vi "读取数据库.vi"(5 "精度(6)":i16=2, 7 "condition":string, 8 "error in (no error)":errorcluster caption="错误输入（无错误）", 9 "database":string="database1.mdb", 10 "显示项":string[](array[string]), 11 "组合框":string(combo)) -> (0 "error out":errorcluster caption="错误输出", 1 "columns":string[](array[string]), 2 "data":variant[][](array[variant]), 3 "表格":string[][](table))   [LabVIEW 2016]
uses:
  <vilib>/Utility/sysdir.llb/System Directory Type.ctl
  <vilib>/addons/database/Connection.llb/DB Tools Open Connec (String).vi
  <vilib>/addons/database/_DB Variant To Data/Database Variant To Data.xnode
  <vilib>/addons/database/NI_Database_API.lvlib
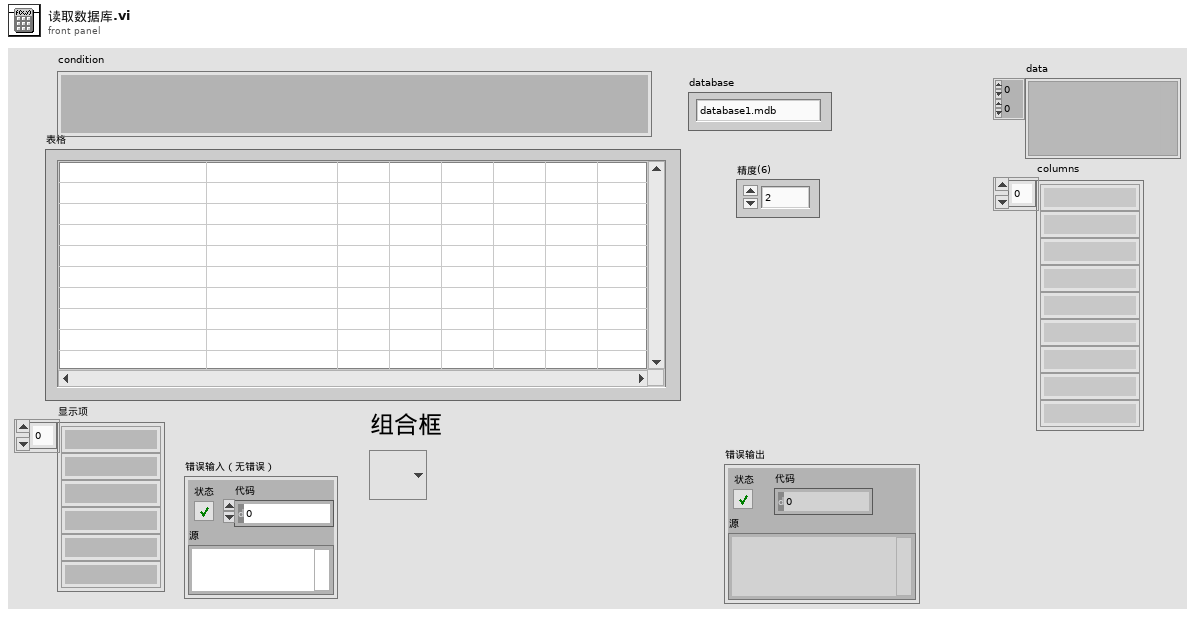
[diagram p1: front panel]
types:
  T1 = typedef "System Directory Type.ctl" = i32
  T2 = typedef "NI_Database_API.lvlib/Conn ObjectReference.ctl" = refnum<k1>
  T3 = typedef "NI_Database_API.lvlib/DB Tools DataTypes.ctl" = enum16{"String", "Long (I32)", "Single (SGL)", "Double (DBL)", "Date/Time", "Binary"}
  T4 = cluster{"name":string, "database data type":T3, "defined size":i32}[]
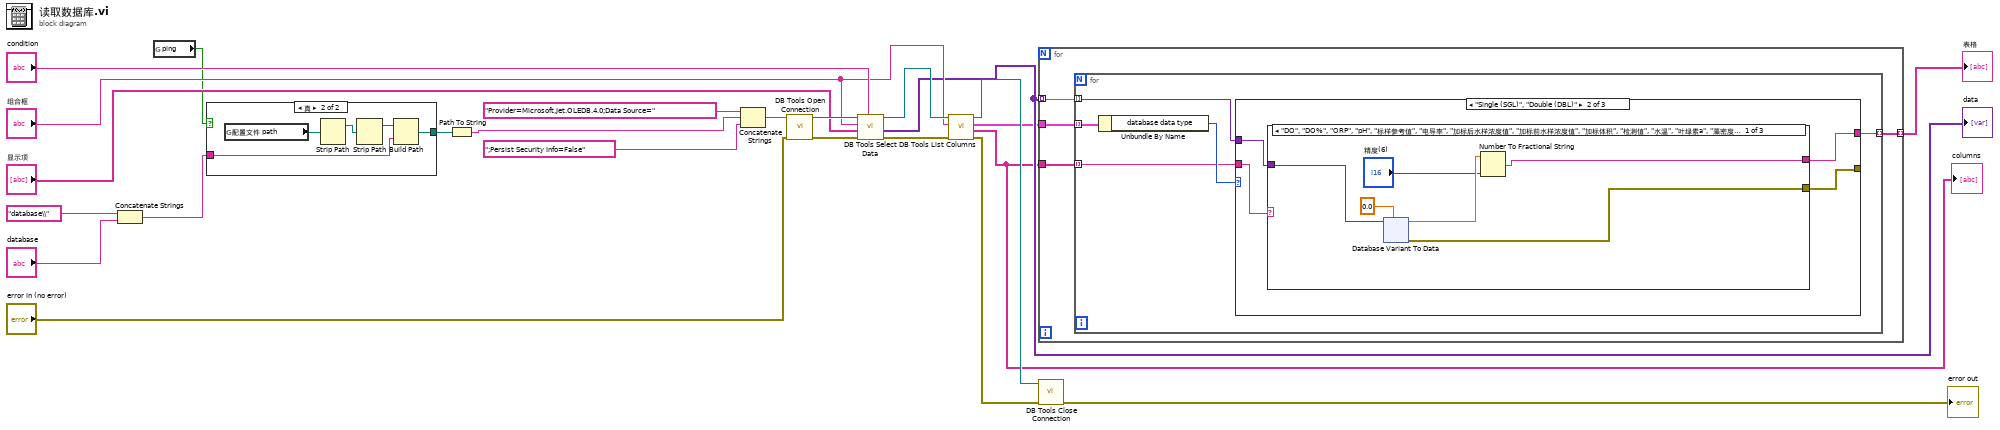
[diagram p0: block diagram]
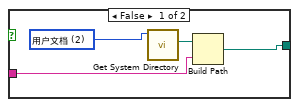
[diagram p2: hidden frame]
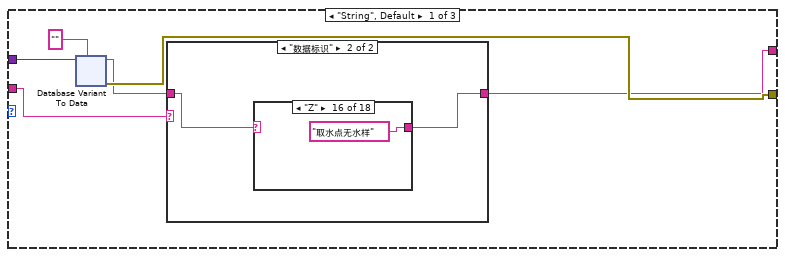
[diagram p3: hidden frame]
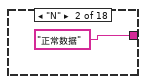
[diagram p6: hidden frame]
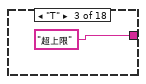
[diagram p7: hidden frame]
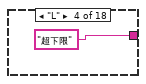
[diagram p8: hidden frame]
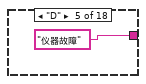
[diagram p9: hidden frame]
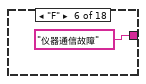
[diagram p10: hidden frame]
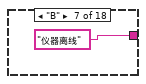
[diagram p11: hidden frame]
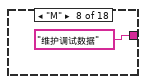
[diagram p12: hidden frame]
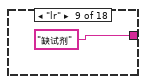
[diagram p13: hidden frame]
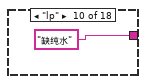
[diagram p14: hidden frame]
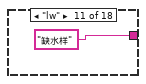
[diagram p15: hidden frame]
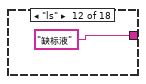
[diagram p16: hidden frame]
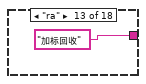
[diagram p17: hidden frame]
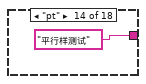
[diagram p18: hidden frame]
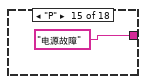
[diagram p19: hidden frame]
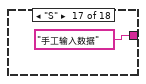
[diagram p20: hidden frame]
diagram:
  n1 = Concatenate Strings("database\\" ("名称或相对路径"), "database") -> (w2:string)
  n2 = global read "ping全局.vi" "ping"() -> (w3:bool)
  n3 = case shown="真" w3 {
    tunnel: w2 -> [w26 w31]
    tunnel: [w25 w29] -> w1
    frame False {
      w27 = T1 2 items=["用户目录"=0, "用户桌面"=1, "用户文档"=2, "用户应用程序数据"=3, "用户设置"=4, "用户临时目录"=5, "公共文档"=6, "公共应用程序数据"=7, "公共设置"=8, "公共缓存"=13, "系统核心库"=9, "系统安装库"=10, "应用程序文件"=11, "启动盘根目录"=12] ("system directory type")
      n4 = call <vilib>:"Get System Directory.vi"("system directory type"=w27) -> ("system directory"=w28:path)  [unwired: 10 in]
      n5 = Build Path(base path=w28, name or relative path=w26) -> (appended path=w25:path)
    }
    frame True {
      n6 = global read "ping全局.vi" "配置文件 path"() -> (w33:path)
      n7 = Strip Path(path=w33) -> (stripped path=w32:path)  [unwired: 1 out]
      n8 = Strip Path(path=w32) -> (stripped path=w30:path)  [unwired: 1 out]
      n9 = Build Path(base path=w30, name or relative path=w31) -> (appended path=w29:path)
    }
  }
  n10 = Path To String(path=w1) -> (string=w12:string)
  n11 = Concatenate Strings("Provider=Microsoft.Jet.OLEDB.4.0;Data Source=", w12, ";Persist Security Info=False") -> (w11:string)
  n12 = call-poly <vilib>:"DB Tools Open Connection.vi"("error in (no error)"="error in (no error)", "connection information"=w11) -> ("error out"=w23:errorcluster, "connection reference"=w24:T2)  [unwired: 6 in]
  n13 = call <vilib>:"DB Tools Select Data.vi"("condition"="condition", "error in (no error)"=w23, "columns"="显示项", "table"="组合框", "connection reference"=w24) -> ("error out"=w22:errorcluster, "data"=w7:variant[][], "connection reference out"=w19:T2)  [unwired: 1 in]
  "data" <- w7
  n14 = call <vilib>:"DB Tools List Columns.vi"("error in (no error)"=w22, "table"="组合框", "connection reference"=w19) -> ("error out"=w15:errorcluster, "columns"=w4:string[], "column information"=w6:T4, "connection reference out"=w16:T2)  [unwired: 1 in]
  "columns" <- w4
  n15 = for {
    tunnel: w7 -> [w37] mode=indexing
    tunnel: w6 -> [w36]
    tunnel: [w35] -> w5 mode=indexing
    tunnel: w4 -> [w34]
    n16 = for {
      tunnel: w37 -> [w41] mode=indexing
      tunnel: w36 -> [w40] mode=indexing
      tunnel: [w39] -> w35 mode=indexing
      tunnel: w34 -> [w38] mode=indexing
      n17 = Unbundle By Name(w40) -> ("database data type"=w42:T3)
      n18 = case shown="\"Single (SGL)\", \"Double (DBL)\"" w42 {
        tunnel: w41 -> [w48 w105 w233]
        tunnel: [w44 w104 w229] -> w39
        tunnel: [w46 w103 w228] -> _
        tunnel: w38 -> [w43 w102 _]
        frame "String", Default {
          n19 = xnode "Database Variant To Data"("database variant"=w48, "type"="") -> ("data"=w45:string, "error out"=w46:errorcluster)  [unwired: 1 in]
          n20 = case shown="\"数据标识\"" w43 {
            tunnel: w45 -> [w49 w51]
            tunnel: [w49 w50] -> w44
            frame Default {
            }
            frame "数据标识" {
              n21 = case shown="\"Z\"" w51 {
                selector: w51 -> [w52 _ _ _ _ _ _ _ _ _ _ _ _ _ _ _ _ _]
                tunnel: [w52 "正常数据" "超上限" "超下限" "仪器故障" "仪器通信故障" "仪器离线" "维护调试数据" "缺试剂" "缺纯水" "缺水样" "缺标液" "加标回收" "平行样测试" "电源故障" "取水点无水样" "手工输入数据" "手动测试数据"] -> w50
                frame Default {
                }
                frame "N" {
                }
                frame "T" {
                }
                frame "L" {
                }
                frame "D" {
                }
                frame "F" {
                }
                frame "B" {
                }
                frame "M" {
                }
                frame "lr" {
                }
                frame "lp" {
                }
                frame "lw" {
                }
                frame "ls" {
                }
                frame "ra" {
                }
                frame "pt" {
                }
                frame "P" {
                }
                frame "Z" {
                }
                frame "S" {
                }
                frame "hd" {
                }
              }
            }
          }
        }
        frame "Single (SGL)", "Double (DBL)" {
          n22 = case shown="\"DO\", \"DO%\", \"ORP\", \"pH\", \"标样参考值\", \"电导率\", \"加标后水样浓度值\", \"加标前水样浓度值\", \"加标体积\", \"检测值\", \"水温\", \"叶绿素a\", \"藻密度\"" w102 {
            selector: w102 -> [_ _ w184]
            tunnel: w105 -> [w111 w149 w187]
            tunnel: [w109 w147 w182] -> w104
            tunnel: [w106 w144 w185] -> w103
            frame "DO", "DO%", "ORP", "pH", "标样参考值", "电导率", "加标后水样浓度值", "加标前水样浓度值", "加标体积", "检测值", "水温", "叶绿素a", "藻密度" {
              n23 = xnode "Database Variant To Data"("database variant"=w111, "type"=0.0) -> ("data"=w110:dbl, "error out"=w106:errorcluster)  [unwired: 1 in]
              n24 = Number To Fractional String(number=w110, precision (6)="精度(6)") -> (F-format string=w109:string)  [unwired: 2 in]
            }
            frame "F0", "f1", "f2", "f3", "f4", "f5", "f6", "f7", "x", "信号值" {
              n25 = xnode "Database Variant To Data"("database variant"=w149, "type"=0.0) -> ("data"=w148:dbl, "error out"=w144:errorcluster)  [unwired: 1 in]
              n26 = Format Into String(format string="%#.4f" ("格式字符串"), w148) -> (resulting string=w147:string)  [unwired: 2 in, 1 out]
            }
            frame Default {
              n27 = xnode "Database Variant To Data"("database variant"=w187, "type"=0.0) -> ("data"=w183:dbl, "error out"=w185:errorcluster)  [unwired: 1 in]
              n28 = case shown="默认" w184 {
                tunnel: w183 -> [w189 w195]
                tunnel: [w188 w191] -> w182
                frame Default {
                  n29 = Format Into String(format string="%#.2f" ("格式字符串"), w189) -> (resulting string=w188:string)  [unwired: 2 in, 1 out]
                }
                frame "量程" {
                  n30 = Equal To 0?(x=w195) -> (x = 0?=w194:bool)
                  n31 = Select(t="低量程" ("格式字符串"), s=w194, f="高量程" ("格式字符串")) -> (s? t:f=w191:string)
                }
              }
            }
          }
        }
        frame "Date/Time" {
          n32 = xnode "Database Variant To Data"("database variant"=w233, "type"=timestamp(0 s since 1904-01-01) ("当前时间")) -> ("data"=w232:timestamp, "error out"=w228:errorcluster)  [unwired: 1 in]
          n33 = Format Date/Time String(time format string (%c)="%y/%m/%d %H:%M:%S" ("时间格式字符串(%c)"), seconds (now)=w232) -> (date/time string=w229:string)  [unwired: 1 in]
        }
      }
    }
  }
  "表格" <- w5
  n34 = call <vilib>:"DB Tools Close Connection.vi"("error in (no error)"=w15, "connection reference"=w16) -> ("error out"=→"error out":errorcluster)  [unwired: 5 in]
